vi "Swerve Math.vi"(9 "Yaw":dbl=88.3, 10 "Rot. Point Y":dbl, 11 "Rot. Point X":dbl) -> (3 "Swerve Math Ouput":dbl[](array[numeric])=[0.0, 0.0, 0.0, 0.0, 0.0, 10.75, 16.677080080157918, 12.75])   [LabVIEW 2018]
uses:
  Drive Train Global.vi
  Robot Information/Robot Information Global.vi
  <vilib>/addons/control/pid/pid.llb/PID (DBL).vi
  <vilib>/addons/control/pid/NI_PID_pid.lvlib
panel:
  in  "PID gains":T1={"proportional gain (Kc)"=0.03, "integral time (Ti, min)"=0.0, "derivative time (Td, min)"=0.0} {"derivative time (Td, min)" format="%.3f"; "integral time (Ti, min)" format="%.3f"; "proportional gain (Kc)" format="%.3f"}
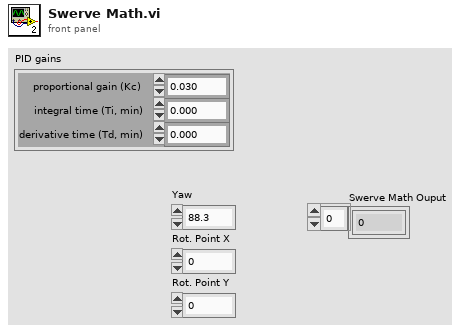
[diagram p1: front panel]
types:
  T1 = cluster{"proportional gain (Kc)":dbl, "integral time (Ti, min)":dbl, "derivative time (Td, min)":dbl}
  T2 = cluster{"Rollover":dbl, "Yaw":dbl, "Cont Yaw":dbl}
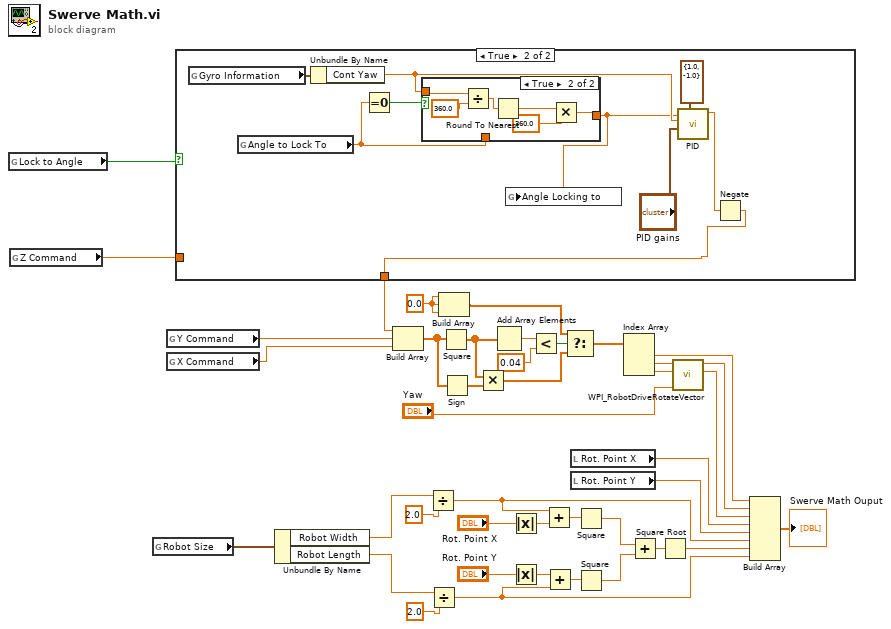
[diagram p0: block diagram]
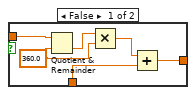
[diagram p3: hidden frame]
diagram:
  w11 = 0.0 ("element")
  n1 = global read "Drive Train Global.vi" "Lock to Angle"() -> (w1:bool)
  n2 = global read "Drive Train Global.vi" "Z Command"() -> (w2:dbl)
  n3 = global read "Robot Information Global.vi" "Robot Size"() -> (w18:cluster{"Robot Width":dbl, "Robot Length":dbl})
  n4 = global read "Drive Train Global.vi" "Y Command"() -> (w5:dbl)
  n5 = global read "Drive Train Global.vi" "X Command"() -> (w19:dbl)
  n6 = case shown="True" w1 {
    tunnel: [w42 w45] -> w3
    tunnel: w2 -> [w42 _]
    frame False {
    }
    frame True {
      n7 = global read "Drive Train Global.vi" "Gyro Information"() -> (w51:T2)
      n8 = global read "Drive Train Global.vi" "Angle to Lock To"() -> (w44:dbl)
      n9 = Unbundle By Name(w51) -> ("Cont Yaw"=w48:dbl)
      n10 = Equal To 0?(x=w44) -> (x = 0?=w43:bool)
      n11 = case shown="True" w43 {
        tunnel: w48 -> [w57 w63]
        tunnel: w44 -> [w56 _]
        tunnel: [w55 w58] -> w47
        frame False {
          w53 = 360.0 ("y")
          n12 = Quotient & Remainder(x=w57, y=w53) -> (floor(x/y)=w54:dbl)  [unwired: 1 out]
          n13 = Multiply(x=w54, y=w53) -> (x*y=w52:dbl)
          n14 = Add(x=w52, y=w56) -> (x+y=w55:dbl)
        }
        frame True {
          n15 = Divide(x=w63, y=360.0) -> (x/y=w61:dbl)
          n16 = Round To Nearest(number=w61) -> (nearest integer value=w60:dbl)
          n17 = Multiply(x=w60, y=360.0) -> (x*y=w58:dbl)
        }
      }
      n18 = global write "Drive Train Global.vi" "Angle Locking to"(w47) -> ()
      n19 = call-poly <vilib>:"PID.vi"("output range"=cluster{"output high":dbl, "output low":dbl} {"output high"=1.0, "output low"=-1.0}, "PID gains"="PID gains", "process variable"=w48, "setpoint"=w47) -> ("output"=w46:dbl)  [unwired: 6 in, 1 out]
      n20 = Negate(x=w46) -> (-x=w45:dbl)
    }
  }
  n21 = Unbundle By Name(w18) -> ("Robot Width"=w16:dbl, "Robot Length"=w17:dbl)
  n22 = Build Array(w3, w5, w19) -> (w7:dbl[])
  n23 = Divide(x=w16, y=2.0) -> (x/y=w27:dbl)
  n24 = Divide(x=w17, y=2.0) -> (x/y=w25:dbl)
  n25 = Build Array(w11, w11, w11) -> (w12:dbl[])
  n26 = Square(x=w7) -> (x^2=w9:dbl[])
  n27 = Sign(1:w7) -> (0:w10:dbl[])
  n28 = Multiply(x=w9, y=w10) -> (x*y=w8:dbl[])
  n29 = Add Array Elements(numeric array=w9) -> (sum=w15:dbl)
  n30 = Absolute Value(x="Rot. Point X") -> (abs(x)=w41:dbl)
  n31 = Absolute Value(x="Rot. Point Y") -> (abs(x)=w39:dbl)
  n32 = Less?(x=w15, y=0.04 ("x")) -> (x < y?=w13:bool)
  n33 = Add(x=w27, y=w41) -> (x+y=w40:dbl)
  n34 = Add(x=w39, y=w25) -> (x+y=w38:dbl)
  n35 = Select(t=w12, s=w13, f=w8) -> (s? t:f=w23:dbl[])
  n36 = local read "Rot. Point X"() -> (w29:dbl)
  n37 = local read "Rot. Point Y"() -> (w28:dbl)
  n38 = Square(x=w40) -> (x^2=w36:dbl)
  n39 = Square(x=w38) -> (x^2=w37:dbl)
  n40 = Index Array(array=w23) -> (element #1=w21:dbl, element #2=w24:dbl, element #3=w30:dbl)  [unwired: 3 in]
  n41 = Add(x=w36, y=w37) -> (x+y=w35:dbl)
  n42 = Square Root(x=w35) -> (sqrt(x)=w26:dbl)
  n43 = call <vilib>:"WPI_RobotDriveRotateVector.vi"("Angle"="Yaw", "X"=w30, "Y"=w24) -> ("X'"=w22:dbl, "Y'"=w20:dbl)  [unwired: 7 out]
  n44 = Build Array(w21, w20, w22, w29, w28, w27, w26, w25) -> (→"Swerve Math Ouput":dbl[])
